vi "readFromXML.vi"(8 "error in (no error)":errorcluster, 10 "XML in":string="<Elevation>\n  <degreesAlt>90.10</degreesAlt>\n  <minutesArc>80.10</minutesArc>\n  <secondsArc>70.10</secondsArc>\n</Elevation>", 11 "Elevation in":refnum<class "Elevation.lvclass">) -> (0 "error out":errorcluster, 3 "Elevation out":refnum<class "Elevation.lvclass">)   [LabVIEW 2014, in "TCSDataDefinitions.lvlib" / "TCSCommand.lvlib" / "TargetConfiguration.lvlib" / "Target.lvlib" / "FixedTarget.lvlib" / "Elevation.lvclass"]
uses:
  Elevation.lvclass
  <userlib>/Common/UnitsAndXML/FlattenItemWithUnitToXML/FlattenPlaneAngleToXML/PlaneAngleUnit.ctl
  Elevation.lvclass/Elevation.ctl
  <userlib>/Common/UnitsAndXML/UnitsAndXML.lvlib
  <userlib>/Common/XML/XMLParser/XMLParser.lvclass
panel:
  out "secondsArc":dbl[unit]=0.0003398543904577847
  out "minutesArc":dbl[unit]=0.023300145514124296
  out "degreesAlt":dbl[unit]=1.5725416560468908
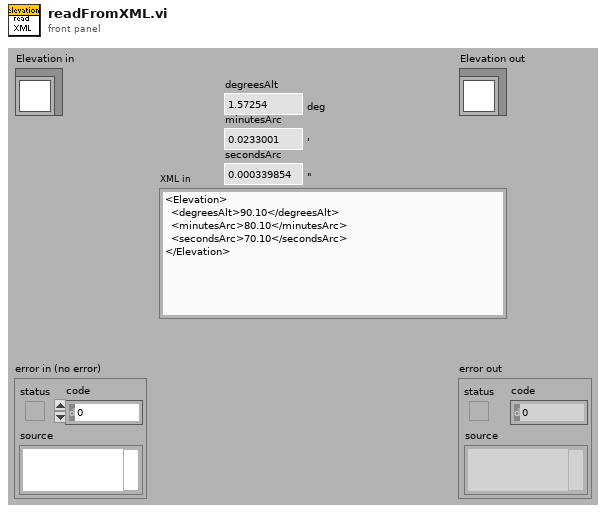
[diagram p1: front panel]
types:
  T1 = typedef "UnitsAndXML.lvlib/PlaneAngleUnit.ctl" = enum16{"rad", "deg", "'", "\""}
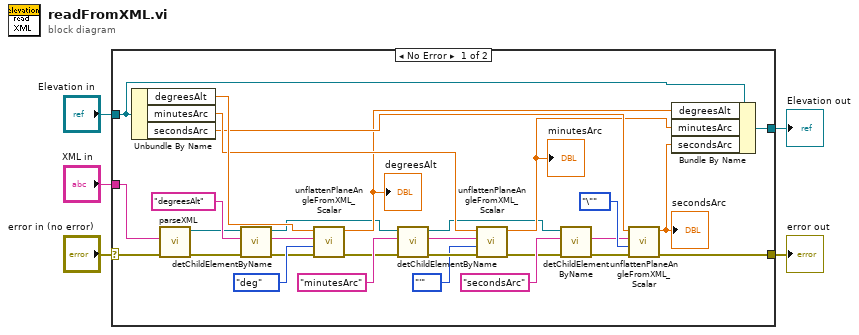
[diagram p0: block diagram]
diagram:
  n1 = case shown="No Error" "error in (no error)" {
    selector: "error in (no error)" -> [w10 w36]
    tunnel: [w11 w36] -> w4
    tunnel: [w12 w35] -> w2
    tunnel: "Elevation in" -> [w13 w35]
    tunnel: "XML in" -> [w9 _]
    frame No Error {
      n2 = Unbundle By Name(w13) -> ("degreesAlt"=w30:dbl[unit], "minutesArc"=w18:dbl[unit], "secondsArc"=w17:dbl[unit])
      n3 = call <userlib>:"parseXML.vi"("error in (no error)"=w10, "XMLString in"=w9) -> ("error out"=w34:errorcluster, "Element out"=w8:refnum<class "XMLParser.lvclass">)  [unwired: 8 in]
      n4 = call <userlib>:"detChildElementByName.vi"("error in (no error)"=w34, "childName"="degreesAlt" ("ChildName"), "Element in"=w8) -> ("error out"=w27:errorcluster, "childXML"=w29:string, "Element out"=w7:refnum<class "XMLParser.lvclass">)  [unwired: 5 in, 1 out]
      n5 = call <userlib>:"unflattenPlaneAngleFromXML_Scalar.vi"("error in (no error)"=w27, "planeAngleUnitInXML"=PlaneAngleUnit."deg", "xmlString"=w29, "planeAngleForType"=w30) -> ("error out"=w26:errorcluster, "planeAngle"=w15:dbl[unit])  [unwired: 6 in]
      "degreesAlt" <- w15
      n6 = call <userlib>:"detChildElementByName.vi"("error in (no error)"=w26, "childName"="minutesArc" ("ChildName"), "Element in"=w7) -> ("error out"=w25:errorcluster, "childXML"=w19:string, "Element out"=w6:refnum<class "XMLParser.lvclass">)  [unwired: 5 in, 1 out]
      n7 = call <userlib>:"unflattenPlaneAngleFromXML_Scalar.vi"("error in (no error)"=w25, "planeAngleUnitInXML"=PlaneAngleUnit."'", "xmlString"=w19, "planeAngleForType"=w18) -> ("error out"=w24:errorcluster, "planeAngle"=w16:dbl[unit])  [unwired: 6 in]
      "minutesArc" <- w16
      n8 = call <userlib>:"detChildElementByName.vi"("error in (no error)"=w24, "childName"="secondsArc" ("ChildName"), "Element in"=w6) -> ("error out"=w23:errorcluster, "childXML"=w20:string)  [unwired: 5 in, 2 out]
      n9 = call <userlib>:"unflattenPlaneAngleFromXML_Scalar.vi"("error in (no error)"=w23, "planeAngleUnitInXML"=PlaneAngleUnit."\"", "xmlString"=w20, "planeAngleForType"=w17) -> ("error out"=w11:errorcluster, "planeAngle"=w14:dbl[unit])  [unwired: 6 in]
      "secondsArc" <- w14
      n10 = Bundle By Name(cluster=w13, "degreesAlt"=w15, "minutesArc"=w16, "secondsArc"=w14) -> (w12:refnum<class "Elevation.lvclass">)
    }
    frame Error {
    }
  }
  "error out" <- w4
  "Elevation out" <- w2
